vi "试剂余量百分比确认.vi"(11 "试剂余量百分比 2":u16 caption="试剂容量") -> (3 "Value":u16)   [LabVIEW 2016, in "斯坦道CODMn新电路板.lvlib"]
panel:
  in  "关闭":bool
  in  "试剂余量百分比":u16=100 format="%.0f %%"
  # "请输入试剂余量百分比"
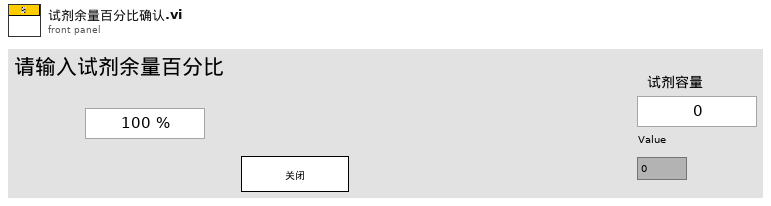
[diagram p1: front panel]
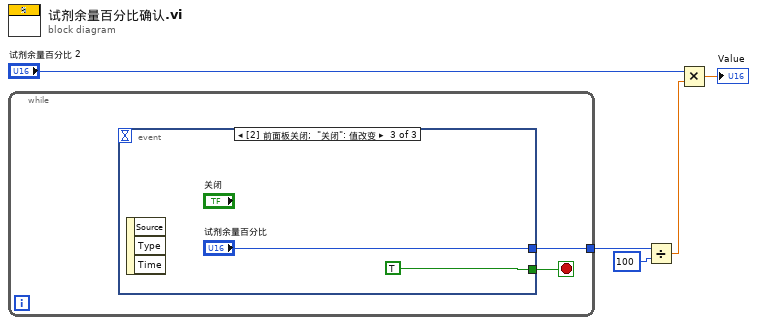
[diagram p0: block diagram]
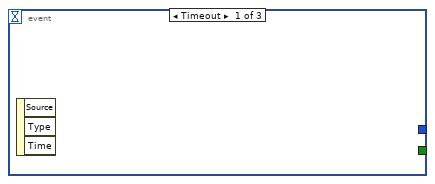
[diagram p2: hidden frame]
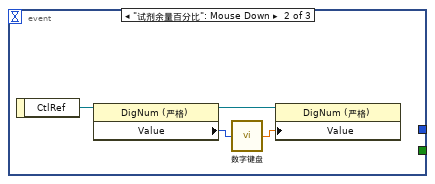
[diagram p3: hidden frame]
diagram:
  n1 = while {
    tunnel: [w6] -> w5
    stop <- w7 stop-if-true
    n2 = event shown="[2] 前面板关闭;  \"关闭\": 值改变" {
      selector: _ -> [_ _ _]
      dyn-events: _ -> [_ _ _]
      timeout: _ -> [_ _ _]
      tunnel: [_ _ TRUE] -> w7
      tunnel: [_ _ "试剂余量百分比"] -> w6
      event Timeout {
        n3 = event-data() -> ()  [unwired: 1 in, 3 out]
      }
      event "试剂余量百分比": Mouse Down {
        n4 = event-data() -> ("CtlRef"=w11:refnum<vi>)  [unwired: 1 in]
        n5 = property class="DigNum (严格)"(reference=w11) -> (reference out=w8:refnum<vi>, "Value"=w10:u16)  [unwired: 1 in, 1 out]
        n6 = call "数字键盘.vi"("OldNumber"=w10) -> ("NewNumber"=w9:dbl)
        n7 = property class="DigNum (严格)"(reference=w8, "Value"=w9) -> ()  [unwired: 1 in, 2 out]
      }
      event Panel Close; "关闭": Value Change {
        n8 = event-data() -> ()  [unwired: 1 in, 3 out]
      }
    }
  }
  n9 = Divide(x=w5, y=u16 100) -> (x/y=w3:dbl)
  n10 = Multiply(x="试剂余量百分比 2", y=w3) -> (x*y=→"Value":dbl)
